vi "HIDRA.vi"() -> ()   [LabVIEW 2015]
uses:
  Control.ctl
  Diagnostics.ctl
  Systems.ctl
  States.ctl
  Data.ctl
  <vilib>/Utility/file.llb/Write Delimited Spreadsheet (DBL).vi
panel:
  out "Pressure":dbl
  out "Systems":T1
  out "Experiment State":T2(ring)
  out "Experiment Purpose":string
  out "Diagnostics":T3
  out "Step Number":i32
  out "Current Step Instructions":string
  in  "Controls":T4
  out "Time Elapsed":string
  out "Current Time":timestamp format="%<%X\n%x>T"
  out "Start Time":timestamp format="%<%X\n%x>T"
  out "Experiment Number":i32
  in  "Exit Button":bool
  out "User Name":string
  # "HIDRA Control System"
  # "User Controls"
  # "Diagnostics"
  # "This button is used for debugging."
  # "Experiment Information"
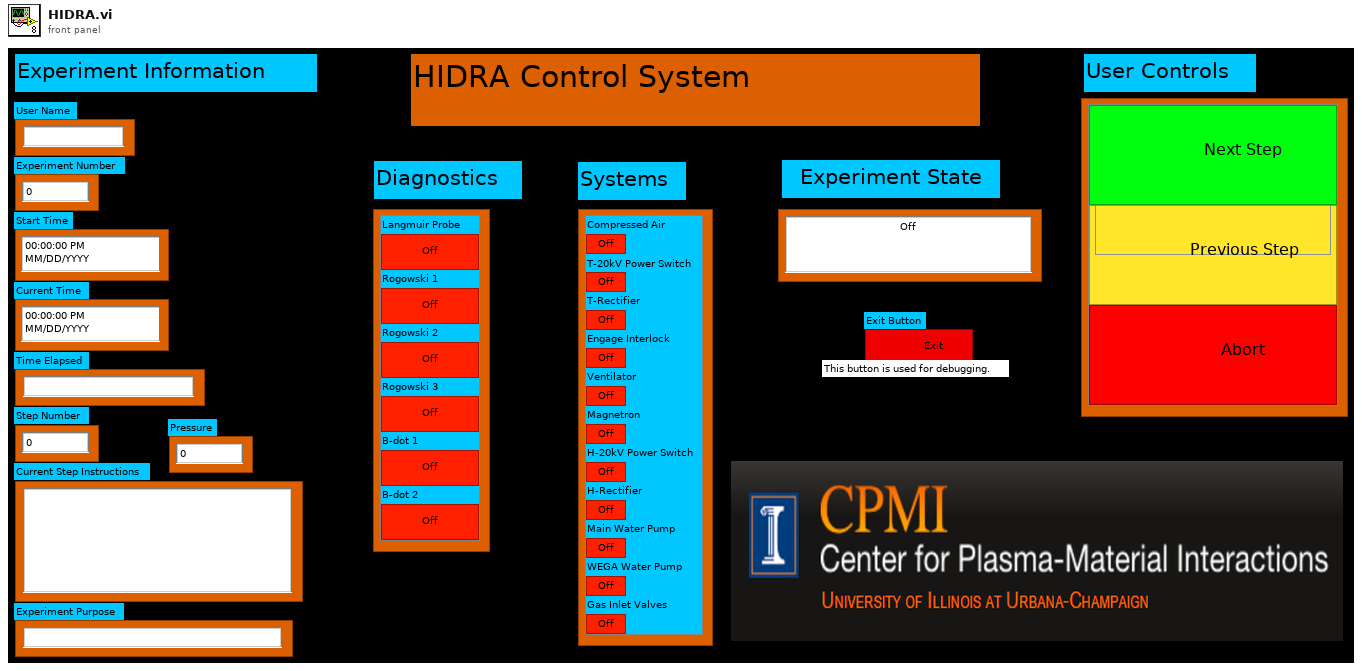
[diagram p1: front panel]
types:
  T1 = typedef "Systems.ctl" = cluster{"Compressed Air":bool, "T-20kV Power Switch":bool, "T-Rectifier":bool, "Engage Interlock":bool, "Ventilator":bool, "Magnetron":bool, "H-20kV Power Switch":bool, "H-Rectifier":bool, "Main Water Pump":bool, "WEGA Water Pump":bool, "Gas Inlet Valves":bool}
  T2 = enum16{"Off", "Setting Up", "Ready", "In Progress", "Shutting Down"}
  T3 = typedef "Diagnostics.ctl" = cluster{"Langmuir Probe":bool, "Rogowski 1":bool, "Rogowski 2":bool, "Rogowski 3":bool, "B-dot 1":bool, "B-dot 2":bool}
  T4 = typedef "Control.ctl" = cluster{"Next Step":bool, "Previous Step":bool, "Abort":bool}
  T5 = typedef "Data.ctl" = cluster{"User Name":string, "Experiment Number":i32, "Start Time":timestamp, "Data":dbl[], "Step Number":i32, "Step Instructions":string, "Diagnostics":T3, "Experiment Purpose":string, "Experiment State":enum16{"Off", "Setting Up", "Ready", "In Progress", "Shutting Down"}, "Systems":T1, "Pressure":dbl, "Field Points":cluster{"System Boolean Fieldpoints":cluster{"Compressed Air":refnum<k21>, "T-20kV Power Switch":refnum<k21>, "T-Rectifier":refnum<k21>, "Engage Interlock":refnum<k21>, "Ventilator":refnum<k21>, "Magnetron":refnum<k21>, "H-20kV Power Switch":refnum<k21>, "H-Rectifier":refnum<k21>, "Main Water Pump":refnum<k21>, "WEGA Water Pump":refnum<k21>, "Gas Inlet Valves":refnum<k21>}}}
  T6 = typedef "States.ctl" = enum16{"1. Initialize", "2. User Information", "3. Experiment Information", "4. Create Data File", "5. Steps for Setup", "6. Gather Data", "7. Write to Data File", "8. Final", "Stop Pressed - Shutdown State"}
  T7 = enum8{"Enabled", "Disabled", "Disabled and Grayed Out"}
  T8 = enum32{"Invalid", "Standard", "Closed", "Hidden", "Minimized", "Maximized"}
  T9 = enum16{"open", "replace", "create", "open or create", "replace or create", "replace or create with confirmation"}
  T10 = enum16{"Always On", "Always Off", "Off While Running"}
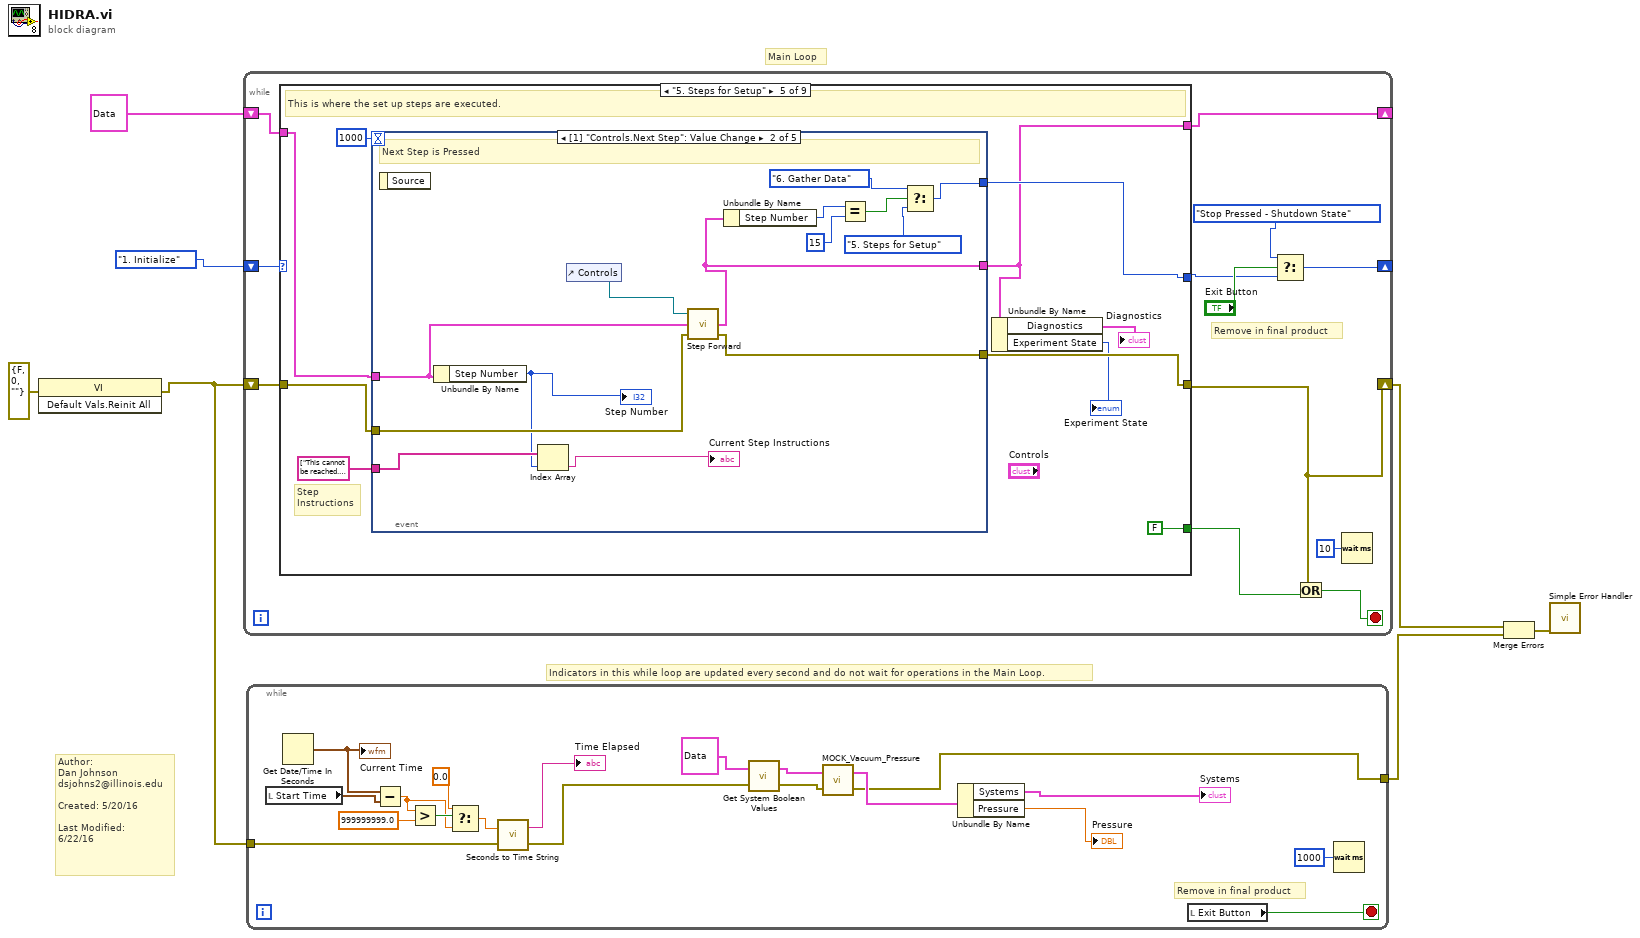
[diagram p0: block diagram]
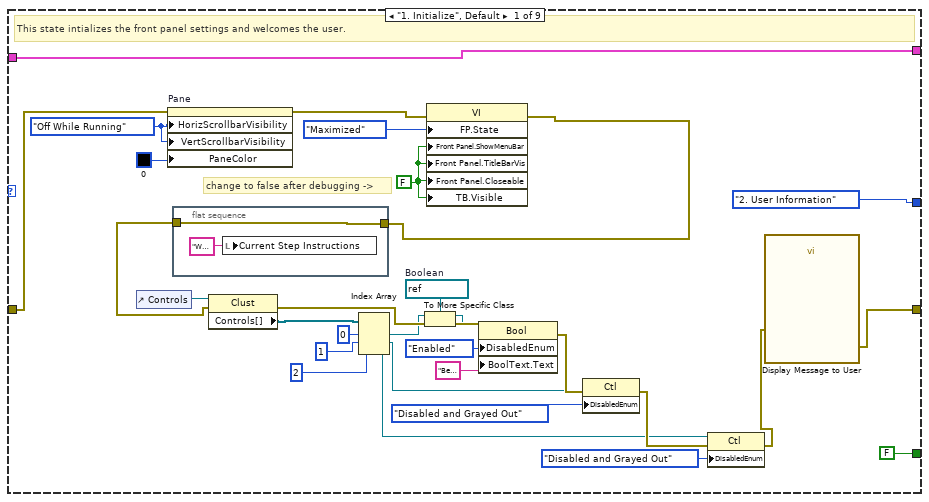
[diagram p2: hidden frame]
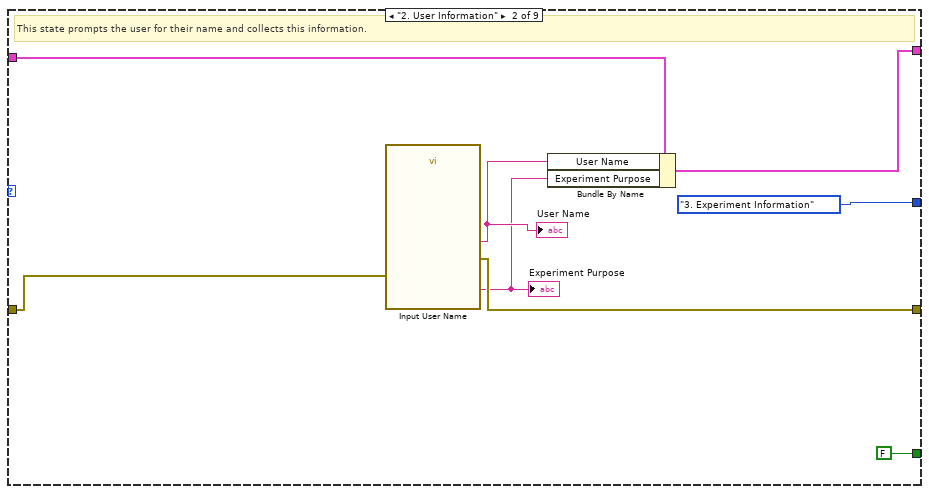
[diagram p3: hidden frame]
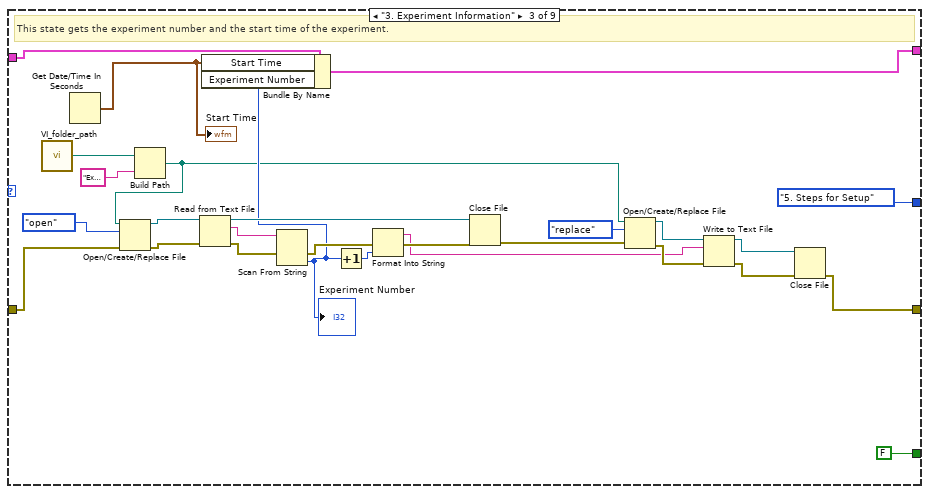
[diagram p4: hidden frame]
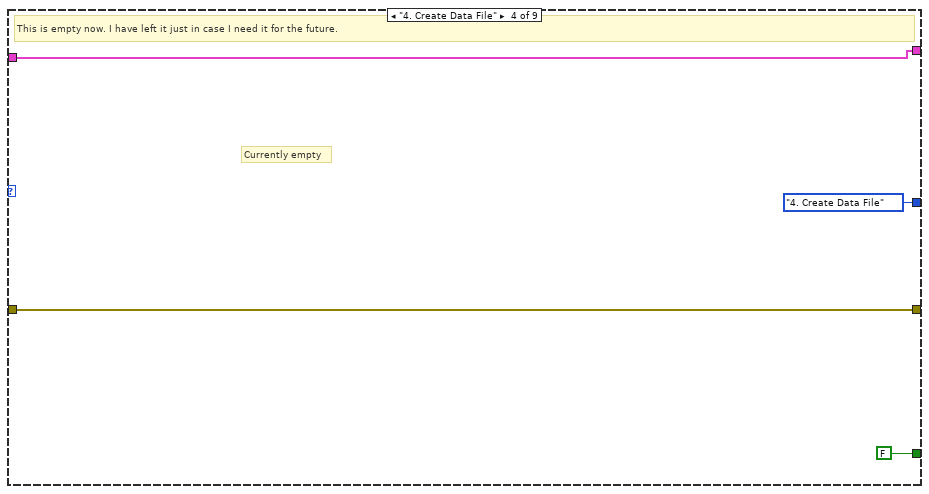
[diagram p5: hidden frame]
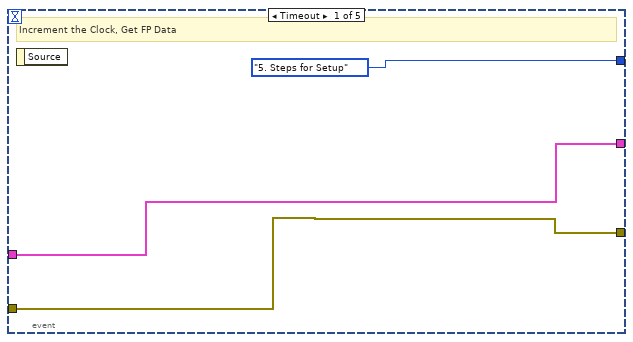
[diagram p6: hidden frame]
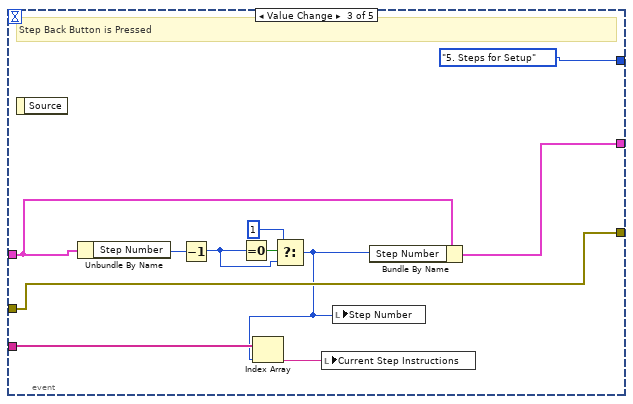
[diagram p7: hidden frame]
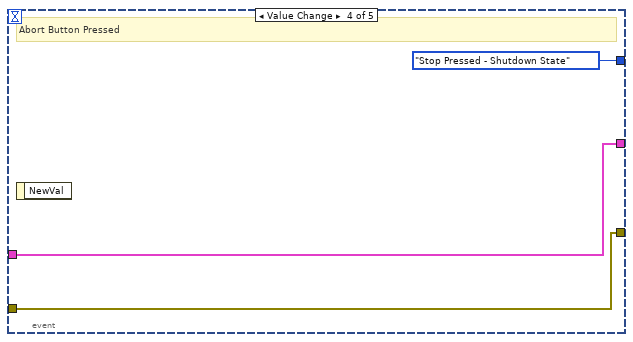
[diagram p8: hidden frame]
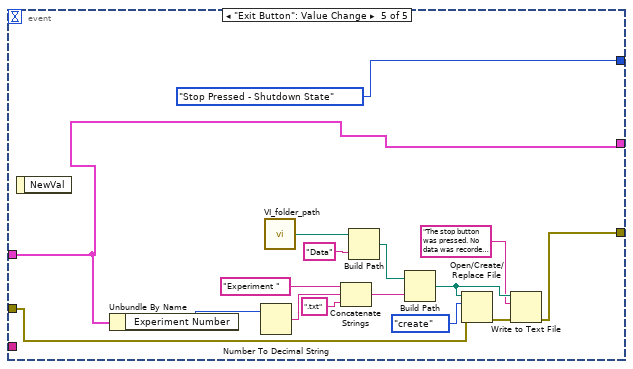
[diagram p9: hidden frame]
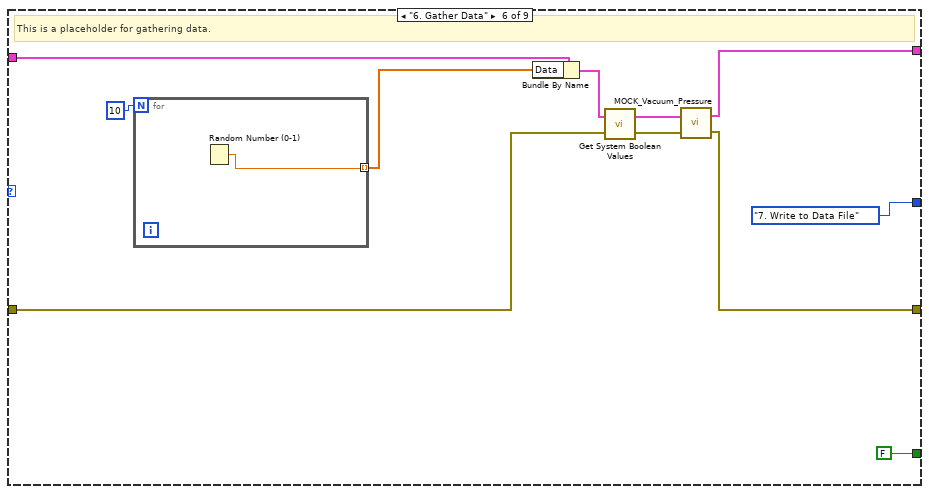
[diagram p10: hidden frame]
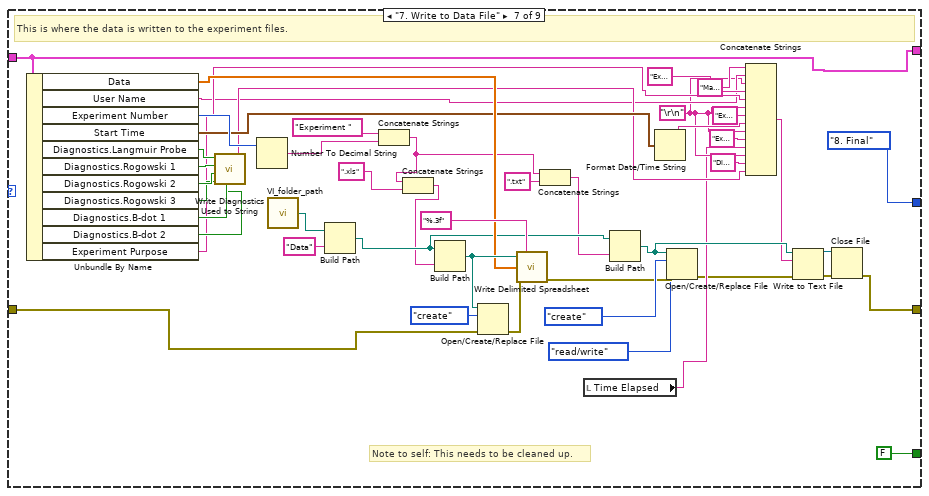
[diagram p11: hidden frame]
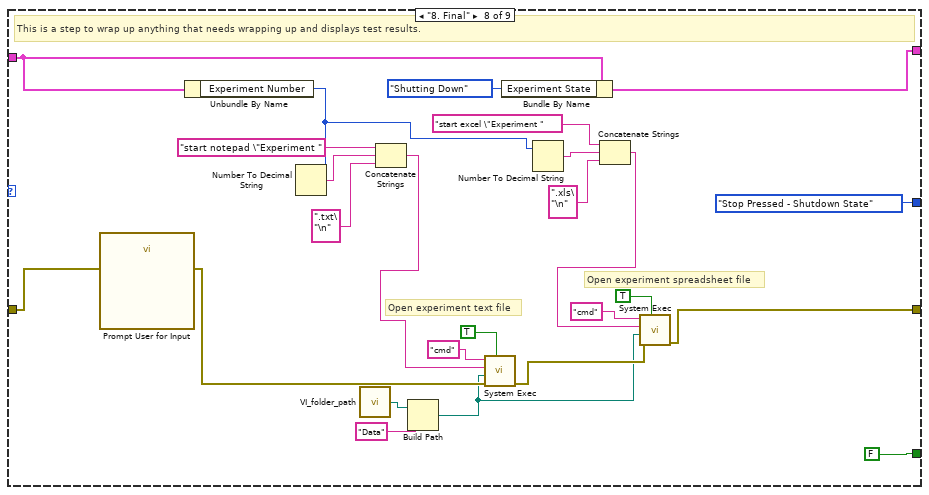
[diagram p12: hidden frame]
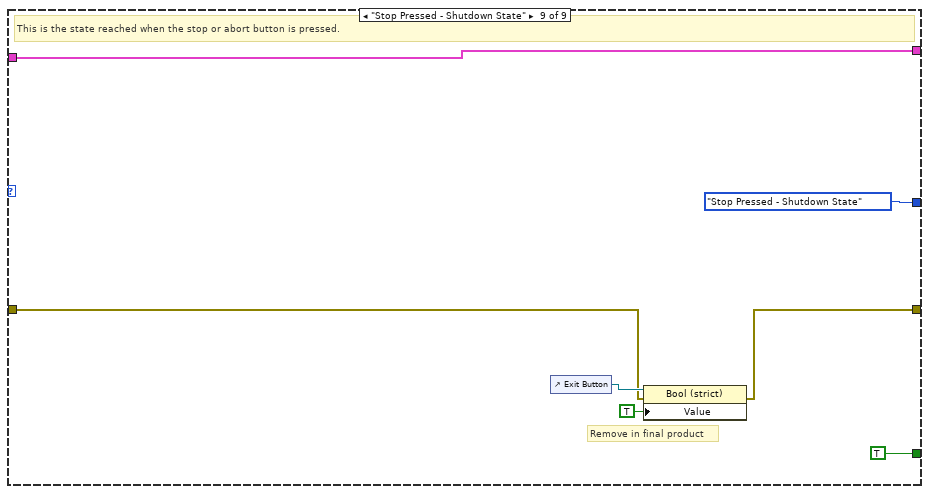
[diagram p13: hidden frame]
diagram:
  # "Main Loop"
  # "Indicators in this while loop are updated every second and do not wait for operations in the Main Loop."
  # "Author:\nDan Johnson\ndsjohns2@illinois.edu\n\nCreated: 5/20/16\n\nLast Modified:\n6/22/16"
  n1 = invoke class="VI" method="Default Vals.Reinit All"(error in=errorcluster {"status"=FALSE, "code"=0, "source"=""} ("error in (no error)")) -> (error out=w2:errorcluster)  [unwired: 2 in, 2 out]
  n2 = while {
    shift-right: [w17] -> _
    shift-left: States."1. Initialize" ("Enum") -> [w10]
    shift-right: [w8] -> _
    shift-left: T5 {"User Name"="", "Experiment Number"=0, "Start Time"=timestamp(0 s since 1904-01-01), "Data"=[], "Step Number"=1, "Step Instructions"="", "Diagnostics"={"Langmuir Probe"=FALSE, "Rogowski 1"=FALSE, "Rogowski 2"=FALSE, "Rogowski 3"=FALSE, "B-dot 1"=FALSE, "B-dot 2"=FALSE}, "Experiment Purpose"="", "Experiment State"=enum."Off", "Systems"={"Compressed Air"=FALSE, "T-20kV Power Switch"=FALSE, "T-Rectifier"=FALSE, "Engage Interlock"=FALSE, "Ventilator"=FALSE, "Magnetron"=FALSE, "H-20kV Power Switch"=FALSE, "H-Rectifier"=FALSE, "Main Water Pump"=FALSE, "WEGA Water Pump"=FALSE, "Gas Inlet Valves"=FALSE}, "Pressure"=0.0, "Field Points"={"System Boolean Fieldpoints"={"Compressed Air"="", "T-20kV Power Switch"="", "T-Rectifier"="", "Engage Interlock"="", "Ventilator"="", "Magnetron"="", "H-20kV Power Switch"="", "H-Rectifier"="", "Main Water Pump"="", "WEGA Water Pump"="", "Gas Inlet Valves"=""}}} ("Data") -> [w18]
    shift-right: [w11] -> w5
    shift-left: w2 -> [w19]
    stop <- w13 stop-if-true
    # "Remove in final product"
    n3 = case shown="\"5. Steps for Setup\"" w10 {
      tunnel: w19 -> [w44 w58 w85 w89 w93 w150 w206 w228 w234]
      tunnel: w18 -> [w50 w56 w65 w90 w100 w158 w196 w218 w238]
      tunnel: [w50 w55 w69 w90 w95 w152 w196 w230 w238] -> w8
      tunnel: [FALSE FALSE FALSE FALSE FALSE FALSE FALSE FALSE TRUE] -> w12
      tunnel: [w43 w57 w64 w89 w97 w149 w170 w221 w233] -> w11
      tunnel: [States."2. User Information" ("Enum") States."3. Experiment Information" ("Enum") States."5. Steps for Setup" ("Enum") States."4. Create Data File" ("Enum") w98 States."7. Write to Data File" ("Enum") States."8. Final" ("Enum") States."Stop Pressed - Shutdown State" ("Enum") States."Stop Pressed - Shutdown State" ("Enum")] -> w9
      frame "1. Initialize", Default {
        w22 = refnum<vi> refnum  # Boolean
        w42 = FALSE
        w46 = T10."Off While Running" ("Vertical Scrollbar Visibility")
        # "change to false after debugging ->"
        # "This state intializes the front panel settings and welcomes the user."
        n4 = control-ref of="Controls"() -> (w40:refnum<vi>)
        n5 = property on="Pane" class="Pane"(error in=w44, "HorizScrollbarVisibility"=w46, "VertScrollbarVisibility"=w46, "PaneColor"=u32 0) -> (error out=w47:errorcluster)  [unwired: 1 in, 1 out]
        n6 = flat-sequence {
          tunnel: [w52] -> w27
          tunnel: w20 -> [w52]
          frame #0 {
            n7 = local write "Current Step Instructions"("Welcome to the Hybrid Illinois Device for Research and Applications (HIDRA)!" ("Current Step Instructions")) -> ()
          }
        }
        n8 = property class="Clust"(reference=w40, error in=w27) -> (error out=w26:errorcluster, "Controls[]"=w29:refnum<vi>[])  [unwired: 1 out]
        n9 = Index Array(array=w29, index #1=0 ("index"), index #2=1 ("index"), index #3=2 ("index")) -> (element #1=w24:refnum<vi>, element #2=w33:refnum<vi>, element #3=w34:refnum<vi>)
        n10 = To More Specific Class(target class=w22, reference=w24, error in=w26) -> (specific class reference=w23:refnum<vi>, error out=w25:errorcluster)
        n11 = property class="VI"(error in=w47, "FP.State"=T8."Maximized" ("Front Panel Window:State"), "Front Panel.ShowMenuBar"=w42, "Front Panel.TitleBarVis"=w42, "Front Panel.Closeable"=w42, "TB.Visible"=w42) -> (error out=w20:errorcluster)  [unwired: 1 in, 1 out]
        n12 = property class="Bool"(reference=w23, error in=w25, "DisabledEnum"=T7."Enabled" ("Disabled"), "BoolText.Text"="Begin Setup Steps" ("Boolean Text.Text")) -> (error out=w35:errorcluster)  [unwired: 1 out]
        n13 = property class="Ctl"(reference=w33, error in=w35, "DisabledEnum"=T7."Disabled and Grayed Out" ("Disabled")) -> (error out=w36:errorcluster)  [unwired: 1 out]
        n14 = property class="Ctl"(reference=w34, error in=w36, "DisabledEnum"=T7."Disabled and Grayed Out" ("Disabled")) -> (error out=w28:errorcluster)  [unwired: 1 out]
        n15 = call "Display Message to User"("error in (no error)"=w28) -> ("error out"=w43:errorcluster)  [unwired: 9 in, 1 out]
      }
      frame "2. User Information" {
        # "This state prompts the user for their name and collects this information."
        n16 = call "Input User Name"("error in (no error)"=w58) -> ("Experiment Purpose"=w53:string, "User Name"=w60:string, "error out"=w57:errorcluster)  [unwired: 15 in, 1 out]
        "User Name" <- w60
        "Experiment Purpose" <- w53
        n17 = Bundle By Name(cluster=w56, "User Name"=w60, "Experiment Purpose"=w53) -> (w55:T5)
      }
      frame "3. Experiment Information" {
        # "This state gets the experiment number and the start time of the experiment."
        n18 = call "VI_folder_path.vi"() -> ("output path"=w63:path)
        n19 = Get Date/Time In Seconds() -> (seconds since 1Jan1904=w67:timestamp)
        "Start Time" <- w67
        n20 = Build Path(base path=w63, name or relative path="Experiment_Number.txt") -> (appended path=w61:path)
        n21 = Open/Create/Replace File(file path (use dialog)=w61, error in=w85, operation (0:open)=T9."open") -> (refnum out=w77:refnum<file>, error out=w84:errorcluster)  [unwired: 3 in, 1 out]
        n22 = Read from Text File(file (use dialog)=w77, error in=w84) -> (refnum out=w76:refnum<file>, text=w72:string, error out=w83:errorcluster)  [unwired: 2 in, 1 out]
        n23 = Scan From String(input string=w72, error in=w83) -> (error out=w82:errorcluster, output 1=w68:i32)  [unwired: 3 in, 2 out]
        "Experiment Number" <- w68
        n24 = Bundle By Name(cluster=w65, "Start Time"=w67, "Experiment Number"=w68) -> (w69:T5)
        n25 = Increment(x=w68) -> (x+1=w71:i32)
        n26 = Format Into String(error in=w82, w71) -> (resulting string=w70:string, error out=w81:errorcluster)  [unwired: 2 in]
        n27 = Close File(refnum=w76, error in=w81) -> (error out=w80:errorcluster)  [unwired: 1 out]
        n28 = Open/Create/Replace File(file path (use dialog)=w61, error in=w80, operation (0:open)=T9."replace") -> (refnum out=w75:refnum<file>, error out=w79:errorcluster)  [unwired: 3 in, 1 out]
        n29 = Write to Text File(file (use dialog)=w75, text=w70, error in=w79) -> (refnum out=w74:refnum<file>, error out=w78:errorcluster)  [unwired: 1 in, 1 out]
        n30 = Close File(refnum=w74, error in=w78) -> (error out=w64:errorcluster)  [unwired: 1 out]
      }
      frame "4. Create Data File" {
        # "Currently empty"
        # "This is empty now. I have left it just in case I need it for the future."
      }
      frame "5. Steps for Setup" {
        # "Step\nInstructions"
        # "This is where the set up steps are executed."
        n31 = event shown="[1] \"Controls.Next Step\": Value Change" {
          selector: _ -> [_ _ _ _ _]
          dyn-events: _ -> [_ _ _ _ _]
          timeout: 1000 -> [_ _ _ _ _]
          tunnel: [States."5. Steps for Setup" ("Enum") w109 States."5. Steps for Setup" ("Enum") States."Stop Pressed - Shutdown State" ("Enum") States."Stop Pressed - Shutdown State" ("Enum")] -> w98
          tunnel: [w102 w116 w120 w130 w137] -> w97
          tunnel: w100 -> [w103 w115 w128 w131 w135]
          tunnel: [w103 w113 w127 w131 w135] -> w95
          tunnel: string[] ["This cannot be reached.", "This step sets up the step controls.", "Select the Diagnostics to be used.", "This step checks that exhaust ventillator is operational.", "This step checks that the compressed air pressure is high enough.", "This step checks that the water pressure is high enough.", "This step checks that the interlock is on.", "This step checks that the toroidal power supply is on.", "This step checks that the toroidal rectifier is on.", "This step checks that the helical power supply is on.", "This step checks that the helical rectifier is on.", "This step sets the magnetron to standby mode.", "This step performs a final check to make sure everything is ready.", "This step does the following:\n  -Starts the Ramp Generator\n  -Opens the Gas Valve\n  -Resets the Radiation Detector", "This step is the pulse."] ("array") -> [_ w118 w125 _ _]
          tunnel: w93 -> [w102 w114 w120 w130 w134]
          event Timeout {
            # "Increment the Clock, Get FP Data"
            n32 = event-data() -> ()  [unwired: 1 in, 1 out]
          }
          event Value Change {
            # "Next Step is Pressed"
            n33 = event-data() -> ()  [unwired: 1 in, 1 out]
            n34 = Unbundle By Name(w115) -> ("Step Number"=w106:i32)
            "Step Number" <- w106
            n35 = Index Array(array=w118, index=w106) -> (element=→"Current Step Instructions":string)
            n36 = control-ref of="Controls"() -> (w117:refnum<vi>)
            n37 = call "Step Forward.vi"("error in"=w114, "Data in"=w115, "Step control reference in"=w117) -> ("error out"=w116:errorcluster, "Data out"=w113:T5)  [unwired: 1 out]
            n38 = Unbundle By Name(w113) -> ("Step Number"=w111:i32)
            n39 = Equal?(x=w111, y=15) -> (x = y?=w112:bool)
            n40 = Select(t=States."6. Gather Data", s=w112, f=States."5. Steps for Setup" ("Enum")) -> (s? t:f=w109:T6)
          }
          event Value Change {
            # "Step Back Button is Pressed"
            n41 = event-data() -> ()  [unwired: 1 in, 1 out]
            n42 = Unbundle By Name(w128) -> ("Step Number"=w129:i32)
            n43 = Decrement(x=w129) -> (x-1=w121:i32)
            n44 = Equal To 0?(x=w121) -> (x = 0?=w123:bool)
            n45 = Select(t=1, s=w123, f=w121) -> (s? t:f=w119:i32)
            n46 = Index Array(array=w125, index=w119) -> (element=w126:string)
            n47 = local write "Current Step Instructions"(w126) -> ()
            n48 = local write "Step Number"(w119) -> ()
            n49 = Bundle By Name(cluster=w128, "Step Number"=w119) -> (w127:T5)
          }
          event Value Change {
            # "Abort Button Pressed"
            n50 = event-data() -> ()  [unwired: 1 in, 1 out]
          }
          event "Exit Button": Value Change {
            n51 = event-data() -> ()  [unwired: 1 in, 1 out]
            n52 = Unbundle By Name(w135) -> ("Experiment Number"=w136:i32)
            n53 = Number To Decimal String(number=w136) -> (decimal integer string=w145:string)  [unwired: 1 in]
            n54 = call "VI_folder_path.vi"() -> ("output path"=w133:path)
            n55 = Concatenate Strings("Experiment " ("string"), w145, ".txt" ("string")) -> (w147:string)
            n56 = Build Path(base path=w133, name or relative path="Data") -> (appended path=w143:path)
            n57 = Build Path(base path=w143, name or relative path=w147) -> (appended path=w140:path)
            n58 = Open/Create/Replace File(file path (use dialog)=w140, error in=w134, operation (0:open)=T9."create") -> (error out=w138:errorcluster)  [unwired: 3 in, 2 out]
            n59 = Write to Text File(file (use dialog)=w140, text="The stop button was pressed. No data was recorded.", error in=w138) -> (error out=w137:errorcluster)  [unwired: 1 in, 2 out]
          }
        }
        n60 = Unbundle By Name(w95) -> ("Diagnostics"=→"Diagnostics":T3, "Experiment State"=→"Experiment State":T2)
      }
      frame "6. Gather Data" {
        # "This is a placeholder for gathering data."
        n61 = for {
          N: 10 -> [_]
          tunnel: [w160] -> w157 mode=indexing
          n62 = Random Number (0-1)() -> (number: 0 to 1=w160:dbl)
        }
        n63 = Bundle By Name(cluster=w158, "Data"=w157) -> (w154:T5)
        n64 = call "Get System Boolean Values.vi"("error in"=w150, "Data in"=w154) -> ("error out"=w151:errorcluster, "Data out"=w153:T5)
        n65 = call "MOCK_Vacuum_Pressure.vi"("error constant"=w151, "Data"=w153) -> ("error constant 2"=w149:errorcluster, "Data 2"=w152:T5)
      }
      frame "7. Write to Data File" {
        w164 = "\r\n"
        # "Note to self: This needs to be cleaned up."
        # "This is where the data is written to the experiment files."
        n66 = Unbundle By Name(w196) -> ("Data"=w195:dbl[], "User Name"=w165:string, "Experiment Number"=w197:i32, "Start Time"=w183:timestamp, "Diagnostics.Langmuir Probe"=w178:bool, "Diagnostics.Rogowski 1"=w177:bool, "Diagnostics.Rogowski 2"=w176:bool, "Diagnostics.Rogowski 3"=w175:bool, "Diagnostics.B-dot 1"=w174:bool, "Diagnostics.B-dot 2"=w173:bool, "Experiment Purpose"=w167:string)
        n67 = call "Write Diagnostics Used to String.vi"("Boolean 6"=w173, "Boolean 5"=w174, "Boolean 4"=w175, "Boolean 3"=w176, "Boolean 2"=w177, "Boolean"=w178) -> ("String"=w171:string)
        n68 = Number To Decimal String(number=w197) -> (decimal integer string=w200:string)  [unwired: 1 in]
        n69 = call "VI_folder_path.vi"() -> ("output path"=w163:path)
        n70 = Build Path(base path=w163, name or relative path="Data") -> (appended path=w191:path)
        n71 = Concatenate Strings("Experiment " ("string"), w200) -> (w188:string)
        n72 = Concatenate Strings(w188, ".xls" ("string")) -> (w189:string)
        n73 = Build Path(base path=w191, name or relative path=w189) -> (appended path=w201:path)
        n74 = Open/Create/Replace File(file path (use dialog)=w201, error in=w206, operation (0:open)=T9."create") -> (error out=w202:errorcluster)  [unwired: 3 in, 2 out]
        n75 = call-poly <vilib>:"Write Delimited Spreadsheet.vi"("file path (dialog if empty)"=w201, "format (%.3f)"="%.3f", "1D data"=w195, "error in (no error)"=w202) -> ("error out"=w193:errorcluster)  [unwired: 10 in, 1 out]
        n76 = Concatenate Strings(w188, ".txt" ("string")) -> (w186:string)
        n77 = local read "Time Elapsed"() -> (w162:string)
        n78 = Build Path(base path=w191, name or relative path=w186) -> (appended path=w172:path)
        n79 = Format Date/Time String(seconds (now)=w183) -> (date/time string=w181:string)  [unwired: 2 in]
        n80 = Open/Create/Replace File(file path (use dialog)=w172, error in=w193, operation (0:open)=T9."create", access (0:read/write)=enum16{"read/write", "read-only", "write-only"}."read/write") -> (error out=w161:errorcluster)  [unwired: 2 in, 2 out]
        n81 = Concatenate Strings("Machine Operator(s): " ("string"), w165, w164, "Experiment Purpose: " ("string"), w167, w164, "Experiment Start Time: " ("string"), w181, w164, "Experiment Time Elapsed: " ("string"), w162, w164, "Diagnostics Used: " ("string"), w171) -> (w169:string)
        n82 = Write to Text File(file (use dialog)=w172, text=w169, error in=w161) -> (refnum out=w185:refnum<file>, error out=w184:errorcluster)  [unwired: 1 in, 1 out]
        n83 = Close File(refnum=w185, error in=w184) -> (error out=w170:errorcluster)  [unwired: 1 out]
      }
      frame "8. Final" {
        # "Open experiment spreadsheet file"
        # "Open experiment text file"
        # "This is a step to wrap up anything that needs wrapping up and displays test results."
        n84 = call "Prompt User for Input"("error in (no error)"=w228) -> ("error out"=w227:errorcluster)  [unwired: 17 in, 1 out]
        n85 = Unbundle By Name(w218) -> ("Experiment Number"=w209:i32)
        n86 = Number To Decimal String(number=w209) -> (decimal integer string=w217:string)  [unwired: 1 in]
        n87 = call "VI_folder_path.vi"() -> ("output path"=w220:path)
        n88 = Concatenate Strings("start notepad \"Experiment " ("string"), w217, ".txt\"\n" ("string")) -> (w213:string)
        n89 = Build Path(base path=w220, name or relative path="Data") -> (appended path=w215:path)
        n90 = call <vilib>:"System Exec.vi"("wait until completion? (T)"=TRUE, "error in (no error)"=w227, "working directory"=w215, "standard input"=w213, "command line"="cmd") -> ("error out"=w222:errorcluster)  [unwired: 3 in, 3 out]
        n91 = Bundle By Name(cluster=w218, "Experiment State"=T2."Shutting Down") -> (w230:T5)
        n92 = Number To Decimal String(number=w209) -> (decimal integer string=w212:string)  [unwired: 1 in]
        n93 = Concatenate Strings("start excel \"Experiment " ("string"), w212, ".xls\"\n" ("string")) -> (w208:string)
        n94 = call <vilib>:"System Exec.vi"("wait until completion? (T)"=TRUE, "error in (no error)"=w222, "working directory"=w215, "standard input"=w208, "command line"="cmd") -> ("error out"=w221:errorcluster)  [unwired: 3 in, 3 out]
      }
      frame "Stop Pressed - Shutdown State" {
        # "Remove in final product"
        # "This is the state reached when the stop or abort button is pressed."
        n95 = control-ref of="Exit Button"() -> (w236:refnum<vi>)
        n96 = property class="Bool (strict)"(reference=w236, error in=w234, "Value"=TRUE) -> (error out=w233:errorcluster)  [unwired: 1 out]
      }
    }
    n97 = Select(t=States."Stop Pressed - Shutdown State" ("Enum"), s="Exit Button", f=w9) -> (s? t:f=w17:T6)
    n98 = Or(x=w11, y=w12) -> (x .or. y?=w13:bool)
    n99 = Wait (ms)(milliseconds to wait=u32 10) -> ()  [unwired: 1 out]
  }
  n100 = while {
    tunnel: [w251] -> w4
    tunnel: w2 -> [w240]
    stop <- w253 stop-if-true
    # "Remove in final product"
    n101 = local read "Start Time"() -> (w248:timestamp)
    n102 = Get Date/Time In Seconds() -> (seconds since 1Jan1904=w249:timestamp)
    "Current Time" <- w249
    n103 = Subtract(x=w249, y=w248) -> (x-y=w242:dbl)
    n104 = Greater?(x=w242, y=999999999.0) -> (0:w244:bool)
    n105 = Select(t=0.0, s=w244, f=w242) -> (s? t:f=w243:dbl)
    n106 = call "Seconds to Time String.vi"("error in"=w240, "Seconds in"=w243) -> ("error out"=w250:errorcluster, "String"=→"Time Elapsed":string)
    n107 = call "Get System Boolean Values.vi"("error in"=w250, "Data in"=T5 {"User Name"="", "Experiment Number"=0, "Start Time"=timestamp(0 s since 1904-01-01), "Data"=[], "Step Number"=1, "Step Instructions"="", "Diagnostics"={"Langmuir Probe"=FALSE, "Rogowski 1"=FALSE, "Rogowski 2"=FALSE, "Rogowski 3"=FALSE, "B-dot 1"=FALSE, "B-dot 2"=FALSE}, "Experiment Purpose"="", "Experiment State"=enum."Off", "Systems"={"Compressed Air"=FALSE, "T-20kV Power Switch"=FALSE, "T-Rectifier"=FALSE, "Engage Interlock"=FALSE, "Ventilator"=FALSE, "Magnetron"=FALSE, "H-20kV Power Switch"=FALSE, "H-Rectifier"=FALSE, "Main Water Pump"=FALSE, "WEGA Water Pump"=FALSE, "Gas Inlet Valves"=FALSE}, "Pressure"=0.0, "Field Points"={"System Boolean Fieldpoints"={"Compressed Air"="", "T-20kV Power Switch"="", "T-Rectifier"="", "Engage Interlock"="", "Ventilator"="", "Magnetron"="", "H-20kV Power Switch"="", "H-Rectifier"="", "Main Water Pump"="", "WEGA Water Pump"="", "Gas Inlet Valves"=""}}} ("Data")) -> ("error out"=w257:errorcluster, "Data out"=w258:T5)
    n108 = call "MOCK_Vacuum_Pressure.vi"("error constant"=w257, "Data"=w258) -> ("error constant 2"=w251:errorcluster, "Data 2"=w252:T5)
    n109 = Unbundle By Name(w252) -> ("Systems"=→"Systems":T1, "Pressure"=→"Pressure":dbl)
    n110 = local read "Exit Button"() -> (w253:bool)
    n111 = Wait (ms)(milliseconds to wait=u32 1000) -> ()  [unwired: 1 out]
  }
  n112 = Merge Errors(w5, w4) -> (w3:errorcluster)
  n113 = call <vilib>:"Simple Error Handler.vi"("error in (no error)"=w3) -> ()  [unwired: 4 in, 5 out]
